vi "Get Frame-Owner Array.vi"(9 "Diagram":refnum<vi>, 11 "References":refnum<vi>[](array[refnum])) -> (3 "Frames-Owners":T1(array[cluster]))   [LabVIEW 2021, in "NI Measurement Plug-In SDK.lvlib" / "VI Info.lvlib"]
doc: "This vi accepts a reference to a block diagram and an array of structure names. It loops through all instances of those structures found in the diagram, and returns an array of references to every possible frame in that diagram, each paired with a reference to its owner and the class name of the structure."
uses:
  VI Info.lvlib
panel:
  # "GObject"
  # "Owner"
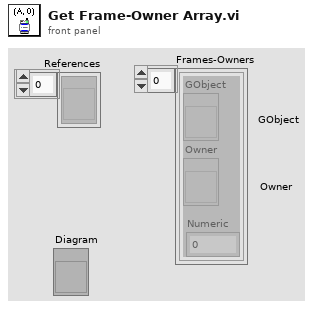
[diagram p1: front panel]
types:
  T1 = cluster{"GObject":refnum<vi>, "Owner":refnum<vi>, "Numeric":dbl}[]
  T2 = cluster{refnum<vi>, "Owner":refnum<vi>, "UID":i32}
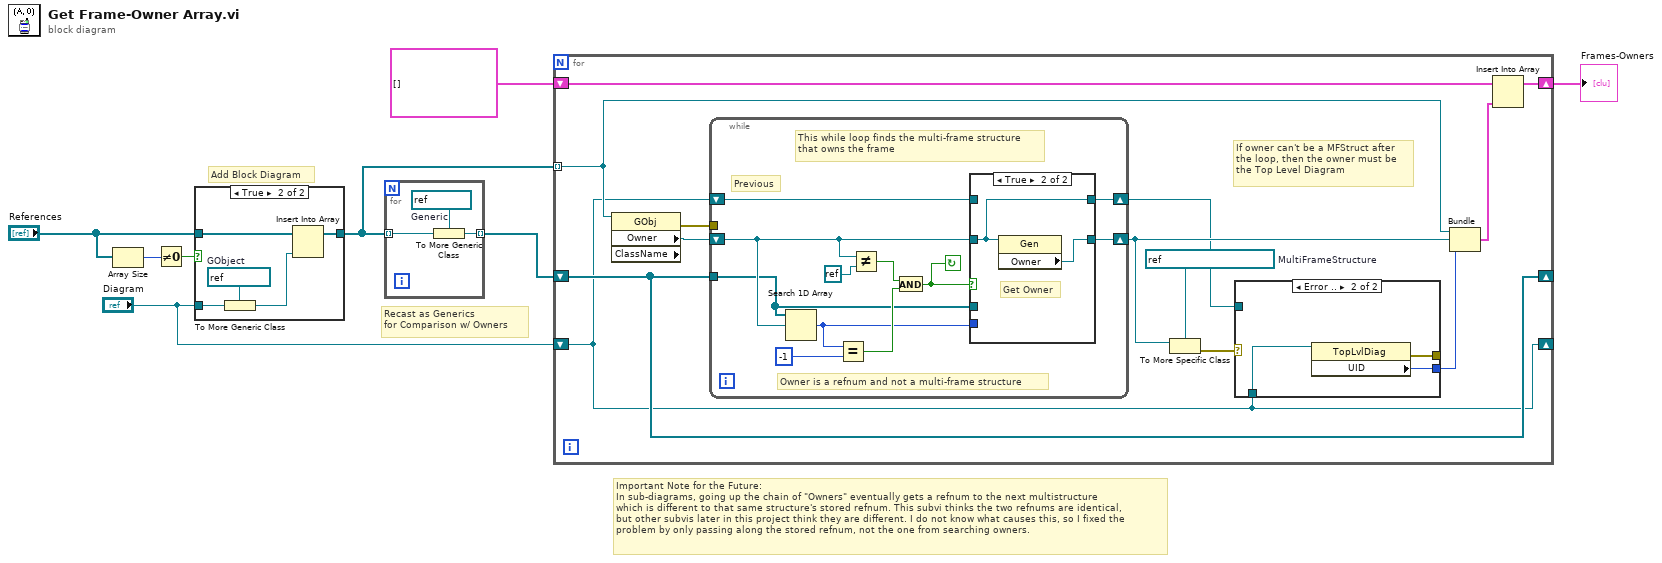
[diagram p0: block diagram]
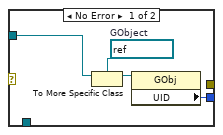
[diagram p3: hidden frame]
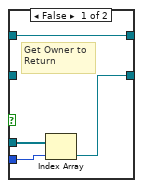
[diagram p4: hidden frame]
diagram:
  # "Recast as Generics\nfor Comparison w/ Owners"
  # "Add Block Diagram"
  # "Important Note for the Future:\nIn sub-diagrams, going up the chain of \"Owners\" eventually gets a refnum to the next multistructure\nwhich is different to that same structure's stored refnum. This subvi thinks the two refnums are identical,\nbut other subvis later in this project think they are different. I do not know what causes this, so I fixed the\nproblem by only passing along the stored refnum, not the one from searching owners."
  n1 = Array Size(array="References") -> (size(s)=w4:i32)
  n2 = Not Equal To 0?(x=w4) -> (x != 0?=w5:bool)
  n3 = case shown="True" w5 {
    tunnel: "References" -> [w9 w14]
    tunnel: "Diagram" -> [_ w12]
    tunnel: [w9 w13] -> w3
    frame False {
    }
    frame True {
      w11 = refnum<vi> refnum  # GObject
      n4 = To More Generic Class(target class=w11, reference=w12) -> (generic class reference=w10:refnum<vi>)
      n5 = Insert Into Array(array=w14, new element=w10) -> (w13:refnum<vi>[])  [unwired: 1 in]
    }
  }
  n6 = for {
    tunnel: w3 -> [w15] mode=indexing
    tunnel: [w17] -> w8 mode=indexing
    w16 = refnum<vi> refnum  # Generic
    n7 = To More Generic Class(target class=w16, reference=w15) -> (generic class reference=w17:refnum<vi>)
  }
  n8 = for {
    shift-right: [w30] -> _
    shift-left: w8 -> [w30]
    shift-right: [w28] -> w6
    shift-left: cluster{refnum<vi>, "Owner":refnum<vi>, i32}[] [] -> [w29]
    tunnel: w3 -> [w22] mode=indexing
    shift-right: [w19] -> _
    shift-left: "Diagram" -> [w19]
    w25 = refnum<vi> refnum  # MultiFrameStructure
    # "If owner can't be a MFStruct after\nthe loop, then the owner must be\nthe Top Level Diagram"
    n9 = property class="GObj" props=["Owner", "ClassName"](reference=w22) -> (error out=w18:errorcluster, "Owner"=w27:refnum<vi>)  [unwired: 1 in, 2 out]
    n10 = while {
      shift-right: [w48] -> w21
      shift-left: w27 -> [w42]
      tunnel: w30 -> [w40]
      shift-right: [w39] -> w20
      shift-left: w19 -> [w38]
      tunnel: w18 -> [_]
      stop <- w43 continue-if-true
      # "This while loop finds the multi-frame structure\nthat owns the frame"
      # "Owner is a refnum and not a multi-frame structure"
      # "Previous"
      n11 = Search 1D Array(1D array=w40, element=w42) -> (index of element=w41:i32)  [unwired: 1 in]
      n12 = Equal?(x=w41, y=-1) -> (x = y?=w44:bool)
      n13 = Not Equal?(x=w42, y=refnum<k0> refnum) -> (x != y?=w46:bool)
      n14 = And(x=w46, y=w44) -> (x .and. y?=w43:bool)
      n15 = case shown="True" w43 {
        tunnel: w42 -> [_ w53]
        tunnel: [w50 w54] -> w48
        tunnel: w41 -> [w52 _]
        tunnel: w40 -> [w51 _]
        tunnel: [w49 w53] -> w39
        tunnel: w38 -> [w49 _]
        frame False {
          # "Get Owner to\nReturn"
          n16 = Index Array(array=w51, index=w52) -> (element=w50:refnum<vi>)
        }
        frame True {
          # "Get Owner"
          n17 = property class="Gen"(reference=w53) -> ("Owner"=w54:refnum<vi>)  [unwired: 1 in, 2 out]
        }
      }
    }
    n18 = To More Specific Class(target class=w25, reference=w21) -> (error out=w24:errorcluster)  [unwired: 1 in, 1 out]
    n19 = case shown="Error .." w24 {
      tunnel: [w31 w37] -> w23
      tunnel: w20 -> [w34 _]
      tunnel: w19 -> [_ w36]
      tunnel: [_ w35] -> _
      frame No Error {
        w33 = refnum<vi> refnum  # GObject
        n20 = To More Specific Class(target class=w33, reference=w34) -> (specific class reference=w32:refnum<vi>)  [unwired: 1 in, 1 out]
        n21 = property class="GObj"(reference=w32) -> ("UID"=w31:i32)  [unwired: 1 in, 2 out]
      }
      frame Error {
        n22 = property class="TopLvlDiag"(reference=w36) -> (error out=w35:errorcluster, "UID"=w37:i32)  [unwired: 1 in, 1 out]
      }
    }
    n23 = Bundle(w22, "Owner"=w21, "UID"=w23) -> (w26:T2)  [unwired: 1 in]
    n24 = Insert Into Array(array=w29, new element=w26) -> (w28:cluster{refnum<vi>, "Owner":refnum<vi>, i32}[])  [unwired: 1 in]
  }
  "Frames-Owners" <- w6
